vi "FCE_TS_Action_DefineCustomErrorCodes.vi"(8 "err in":errorcluster) -> (0 "err out":errorcluster)   [LabVIEW 2017]
uses:
  FCE_TS_General_Libs/WL_Libs_V14.25/WL_Error_V14.00.llb/WL_Error_GlobalCodes.gbl.vi
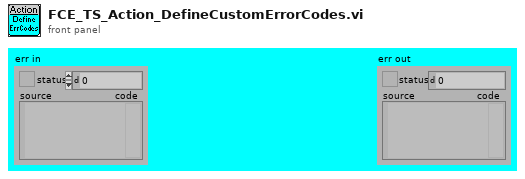
[diagram p1: front panel]
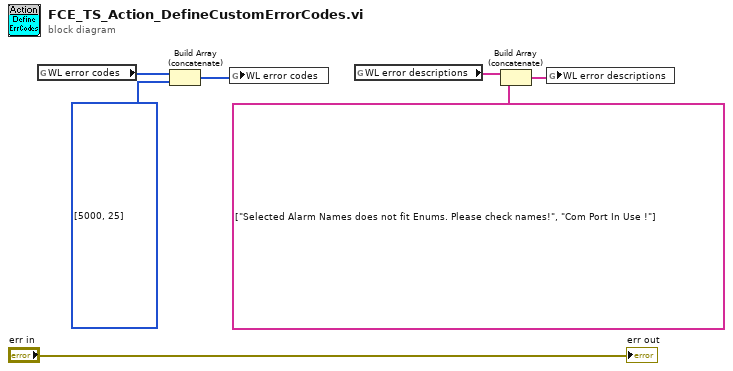
[diagram p0: block diagram]
diagram:
  n1 = global read "WL_Error_GlobalCodes.gbl.vi" "WL error codes"() -> (w6:i32[])
  n2 = Build Array (concatenate)(w6, i32[] [5000, 25] ("element")) -> (w4:i32[])
  n3 = global write "WL_Error_GlobalCodes.gbl.vi" "WL error codes"(w4) -> ()
  n4 = global read "WL_Error_GlobalCodes.gbl.vi" "WL error descriptions"() -> (w2:string[])
  n5 = Build Array (concatenate)(w2, string[] ["Selected Alarm Names does not fit Enums. Please check names!", "Com Port In Use !"] ("array")) -> (w3:string[])
  n6 = global write "WL_Error_GlobalCodes.gbl.vi" "WL error descriptions"(w3) -> ()
  "err out" <- "err in"
